vi "Apply.vi"(8 "error in":errorcluster, 11 "Control Load CFG in":refnum<class "EL Control Load CFG.lvclass">) -> (0 "error out":errorcluster, 3 "Control Load CFG out":refnum<class "EL Control Load CFG.lvclass">)   [LabVIEW 2023, in "EL Control Load CFG.lvclass"]
uses:
  EL Control Load CFG.lvclass
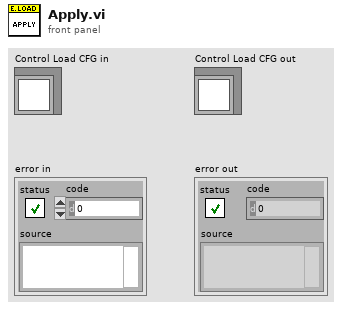
[diagram p1: front panel]
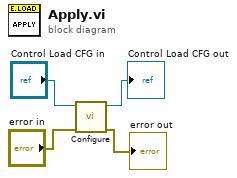
[diagram p0: block diagram]
diagram:
  n1 = call-dynamic "Configure.vi"("error in"="error in", "Control Load CFG in"="Control Load CFG in") -> ("error out"=→"error out":errorcluster, "Control Load CFG out"=→"Control Load CFG out":refnum<class "EL Control Load CFG.lvclass">)  [unwired: 8 in]
